vi "Handle.vi"(7 "Queue in":refnum<class "Queue.lvclass">, 11 "Teardown State in":refnum<class "Teardown State.lvclass">) -> (2 "Destroy?":bool, 5 "Queue out":refnum<class "Queue.lvclass">)   [LabVIEW 2021, in "jettl.lvlib" / "Base Queue.lvlib" / "State.lvlib" / "Teardown State.lvclass"]
uses:
  Teardown State.lvclass
  Queue/Queue.lvclass
  Teardown State.lvclass/Teardown State.ctl
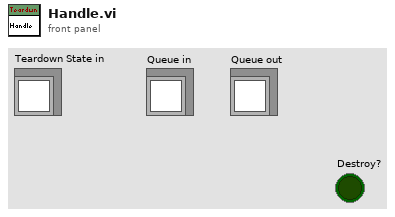
[diagram p1: front panel]
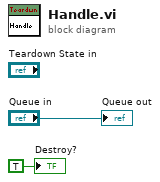
[diagram p0: block diagram]
diagram:
  "Destroy?" <- TRUE ("Destroy?")
  "Queue out" <- "Queue in"
